vi "table line to assembly.vi"(11 "ItemNames":string[](array[string])) -> (3 "assembly definition":T1)   [LabVIEW 2013, in "EIP Tag API editor node.lvclass"]
uses:
  EIP Tag API editor node.lvclass
  <vilib>/NI/TBM Modules/Ethernet IP/configuration/assembly type.ctl
  <vilib>/NI/TBM Modules/Ethernet IP/configuration/assembly definition.ctl
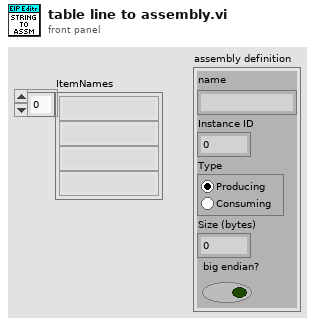
[diagram p1: front panel]
types:
  T1 = typedef "EthernetIP configuration.lvclass/assembly definition.ctl" = cluster{"name":string, "Instance ID":u32, "Type":T2, "Size (bytes)":u32, "big endian?":bool}
  T2 = typedef "EthernetIP configuration.lvclass/assembly type.ctl" = enum32{"Producing", "Consuming"}
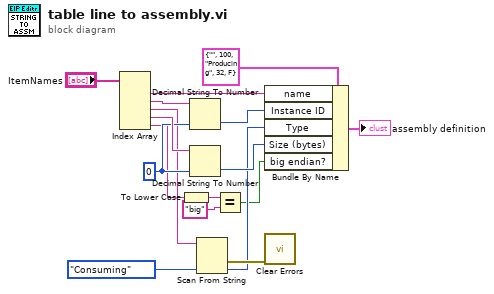
[diagram p0: block diagram]
diagram:
  w9 = u32 0 ("default (0 I32)")
  n1 = Index Array(array="ItemNames") -> (element #1=w14:string, element #2=w13:string, element #3=w5:string, element #4=w12:string, element #5=w4:string)  [unwired: 5 in]
  n2 = To Lower Case(string=w4) -> (all lower case string=w1:string)
  n3 = Decimal String To Number(string=w13, default (0L)=w9) -> (number=w10:u32)  [unwired: 1 in, 1 out]
  n4 = Decimal String To Number(string=w12, default (0L)=w9) -> (number=w11:u32)  [unwired: 1 in, 1 out]
  n5 = Scan From String(input string=w5, default 1=assembly_type."Consuming" ("Type")) -> (error out=w8:errorcluster, output 1=w7:T2)  [unwired: 3 in, 2 out]
  n6 = Equal?(x=w1, y="big") -> (x = y?=w2:bool)
  n7 = Bundle By Name(cluster=T1 {"name"="", "Instance ID"=100, "Type"=enum."Producing", "Size (bytes)"=32, "big endian?"=FALSE} ("assembly definition"), "name"=w14, "Instance ID"=w10, "Type"=w7, "Size (bytes)"=w11, "big endian?"=w2) -> (→"assembly definition":T1)
  n8 = call <vilib>:"Clear Errors.vi"("error in (no error)"=w8) -> ()  [unwired: 6 in, 1 out]
